vi "Lab Panel V5.0.vi"() -> ()   [LabVIEW 2013] (continued)
                        n564 = TDMS Open(6:FALSE, 10:T18."create or replace" ("operation (0:open)"), 11:w898) -> (0:w897:errorcluster, 3:→"TDMS LAB02-1":refnum<k34>)  [unwired: 4 in]
                      }
                      frame #2 {
                        n565 = local read "SET LAB02-1"() -> (w908:T5)
                        n566 = local read "TDMS LAB02-1"() -> (w919:refnum<k34>)
                        n567 = Build Array("Testers Name", "Description", "Set Test Cycles", "T-Rise minutes", "T-Rise Deg C") -> (w909:string[])
                        n568 = Unbundle(w908) -> ("NAME"=w907:string, "DESCRIPTION"=w906:string, "CYCLES"=w905:dbl, "T-RISE mins"=w904:dbl, "T-RISE deg C"=w903:dbl)
                        n569 = Number To Decimal String(number=w905) -> (decimal integer string=w918:string)  [unwired: 1 in]
                        n570 = Number To Decimal String(number=w904) -> (decimal integer string=w917:string)  [unwired: 1 in]
                        n571 = Number To Decimal String(number=w903) -> (decimal integer string=w916:string)  [unwired: 1 in]
                        n572 = Build Array(w907, w906, w918, w917, w916) -> (w915:string[])
                        n573 = TDMS Set Properties(5:w915, 7:w909, 11:w919) -> ()  [unwired: 3 in, 4 out]
                      }
                      frame #3 {
                        n574 = local read "DISP LAB02-1"() -> (w924:T4)
                        n575 = Concatenate Strings("LAB02-1  ", w923) -> (w925:string)
                        n576 = Two Button Dialog(message=w925, 1:w921, 2:w922) -> (T button?=w927:bool)
                        n577 = case shown="True" w927 {
                          tunnel: w924 -> [w934 w935]
                          tunnel: [w934 w935] -> w931
                          tunnel: [w933 w936] -> w930
                          tunnel: [w932 w936] -> w929
                          frame False {
                            n578 = Unbundle(w934) -> ("CYCLE"=w933:dbl, "MINS"=w932:dbl)  [unwired: 1 out]
                          }
                          frame True {
                            w936 = 0.0
                          }
                        }
                        n579 = Bundle(cluster=w931, "CYCLE"=w930, "MINS"=w929, "STATUS"="RUN") -> (w920:T4)
                        n580 = local write "DISP LAB02-1"(w920) -> ()
                      }
                      frame #4 {
                        n581 = local read "SIG LAB02-1"() -> (w939:T2)
                        n582 = local read "TEMP START LAB02-1"() -> (w941:cluster{"TL":dbl, "TN":dbl})
                        n583 = Unbundle(w939) -> ("Tmp Live"=w938:dbl, "Tmp Neut"=w937:dbl)  [unwired: 3 out]
                        n584 = Bundle(cluster=w941, "TL"=w938, "TN"=w937) -> (w940:cluster{"TL":dbl, "TN":dbl})
                        n585 = local write "TEMP START LAB02-1"(w940) -> ()
                      }
                    }
                  }
                }
              }
              event "RUN LAB02-2": Value Change {
                n586 = event-data() -> ("NewVal"=w945:bool)  [unwired: 1 in, 5 out]
                n587 = local write "run lab02-2"(w945) -> ()
                n588 = case shown="True" w945 {
                  tunnel: w951 -> [_ w987]
                  tunnel: w950 -> [_ w986]
                  tunnel: w948 -> [w953 w985]
                  tunnel: w949 -> [_ w984]
                  tunnel: w947 -> [_ w983]
                  tunnel: [w952 w982] -> w946
                  tunnel: w944 -> [_ w981]
                  tunnel: w943 -> [_ w980]
                  tunnel: w942 -> [_ w979]
                  frame False {
                    # "stop test"
                    n589 = stacked-sequence {
                      tunnel: w953 -> [w962 _]
                      tunnel: [w954 _] -> w952
                      frame #0 {
                        n590 = local read "DISP LAB02-2"() -> (w961:T4)
                        n591 = Unbundle(w961) -> ("CYCLE"=w959:dbl, "MINS"=w960:dbl)  [unwired: 1 out]
                        n592 = case shown="\"CYCLE TEST\"" w962 {
                          tunnel: w960 -> [_ _ w969]
                          tunnel: w959 -> [w967 w968 _]
                          tunnel: [w967 w968 w969] -> w958
                          frame "CHART TEST", Default {
                          }
                          frame "CYCLE TEST" {
                          }
                          frame "T-RISE TEST" {
                          }
                        }
                        n593 = local read "TDMS LAB02-2"() -> (w966:refnum<k34>)
                        n594 = Build Array("STOPPED") -> (w963:string[])
                        n595 = Build Array(w958) -> (w957:dbl[])
                        n596 = TDMS Write(0:w966, 5:"TEST RESULT", 7:w963, 9:w957) -> (4:w955:refnum<k34>, 15:w956:errorcluster)  [unwired: 2 in, 2 out]
                        n597 = TDMS Close(8:w956, 11:w955) -> (0:w954:errorcluster)  [unwired: 1 out]
                      }
                      frame #1 {
                        n598 = local read "DISP LAB02-2"() -> (w973:T4)
                        n599 = stacked-sequence {
                          tunnel: "LAB02-2" -> [w975 w977]
                          frame #0 {
                            n600 = call "sub vi - defrag tdms v1.vi"("panel id"=w975) -> ("error out"=w974:errorcluster)  [unwired: 10 in]
                            n601 = local write "data file error"(w974) -> ()
                          }
                          frame #1 {
                            n602 = call "Save data file to network drive v2.vi"("panel id"=w977) -> ("network file save error"=w976:errorcluster)  [unwired: 9 in, 1 out]
                            n603 = local write "RESULT LAB02-2"(FALSE) -> ()
                            n604 = local write "data file error"(w976) -> ()
                          }
                        }
                        n605 = Bundle(cluster=w973, "STATUS"="STOP") -> (w971:T4)  [unwired: 2 in]
                        n606 = local write "DISP LAB02-2"(w971) -> ()
                      }
                    }
                  }
                  frame True {
                    # "start new test and create test file"
                    n607 = stacked-sequence {
                      seq-local: [w988 _ _ _ _] -> [_ w1012 _ _ _]
                      tunnel: w987 -> [w993 _ _ _ _]
                      tunnel: w986 -> [w990 _ _ _ _]
                      tunnel: w985 -> [w1003 _ _ _ _]
                      tunnel: w984 -> [w996 _ _ _ _]
                      tunnel: w983 -> [w991 _ _ _ _]
                      tunnel: [_ w1007 _ _ _] -> w982
                      tunnel: w981 -> [_ _ _ w1033 _]
                      tunnel: w980 -> [_ _ _ w1032 _]
                      tunnel: w979 -> [_ _ _ w1031 _]
                      frame #0 {
                        w989 = "\\"
                        n608 = local read "SET LAB02-2"() -> (w998:T5)
                        n609 = case shown="\"CYCLE TEST\"" w1003 {
                          tunnel: ["L02-2-CHART TEST-" "L02-2-CYCLE TEST-" "L02-2-T-RISE TEST-"] -> w999
                          frame "CHART TEST", Default {
                          }
                          frame "CYCLE TEST" {
                          }
                          frame "T-RISE TEST" {
                          }
                        }
                        n610 = Unbundle(w998) -> ("DESCRIPTION"=w997:string)  [unwired: 4 out]
                        n611 = Concatenate Strings(w993, "\\", w991, w989, w990, w989) -> (w1000:string)
                        n612 = String To Path(string=w1000) -> (path=w1002:path)
                        n613 = Concatenate Strings(w1000, w999, w997, "-", w996, ".tdms") -> (w988:string)
                        n614 = Create Folder(path (use dialog)=w1002) -> (error out=w1001:errorcluster)  [unwired: 2 in, 2 out]
                        n615 = global write "Global 1.vi" "LAB02-2 FILE"(w988) -> ()
                        n616 = call <vilib>:"Clear Errors.vi"("error in (no error)"=w1001) -> ()  [unwired: 6 in, 1 out]
                      }
                      frame #1 {
                        (unwired) FALSE
                        n617 = String To Path(string=w1012) -> (path=w1008:path)
                        n618 = TDMS Open(6:FALSE, 10:T18."create or replace" ("operation (0:open)"), 11:w1008) -> (0:w1007:errorcluster, 3:→"TDMS LAB02-2":refnum<k34>)  [unwired: 4 in]
                      }
                      frame #2 {
                        n619 = local read "SET LAB02-2"() -> (w1018:T5)
                        n620 = local read "TDMS LAB02-2"() -> (w1029:refnum<k34>)
                        n621 = Build Array("Testers Name", "Description", "Set Test Cycles", "T-Rise minutes", "T-Rise Deg C") -> (w1019:string[])
                        n622 = Unbundle(w1018) -> ("NAME"=w1017:string, "DESCRIPTION"=w1016:string, "CYCLES"=w1015:dbl, "T-RISE mins"=w1014:dbl, "T-RISE deg C"=w1013:dbl)
                        n623 = Number To Decimal String(number=w1015) -> (decimal integer string=w1028:string)  [unwired: 1 in]
                        n624 = Number To Decimal String(number=w1014) -> (decimal integer string=w1027:string)  [unwired: 1 in]
                        n625 = Number To Decimal String(number=w1013) -> (decimal integer string=w1026:string)  [unwired: 1 in]
                        n626 = Build Array(w1017, w1016, w1028, w1027, w1026) -> (w1025:string[])
                        n627 = TDMS Set Properties(5:w1025, 7:w1019, 11:w1029) -> ()  [unwired: 3 in, 4 out]
                      }
                      frame #3 {
                        n628 = local read "DISP LAB02-2"() -> (w1034:T4)
                        n629 = Concatenate Strings("LAB02-2  ", w1033) -> (w1035:string)
                        n630 = Two Button Dialog(message=w1035, 1:w1031, 2:w1032) -> (T button?=w1037:bool)
                        n631 = case shown="True" w1037 {
                          tunnel: w1034 -> [w1044 w1045]
                          tunnel: [w1044 w1045] -> w1041
                          tunnel: [w1043 w1046] -> w1040
                          tunnel: [w1042 w1046] -> w1039
                          frame False {
                            n632 = Unbundle(w1044) -> ("CYCLE"=w1043:dbl, "MINS"=w1042:dbl)  [unwired: 1 out]
                          }
                          frame True {
                            w1046 = 0.0
                          }
                        }
                        n633 = Bundle(cluster=w1041, "CYCLE"=w1040, "MINS"=w1039, "STATUS"="RUN") -> (w1030:T4)
                        n634 = local write "DISP LAB02-2"(w1030) -> ()
                      }
                      frame #4 {
                        n635 = local read "SIG LAB02-2"() -> (w1049:T2)
                        n636 = local read "TEMP START LAB02-2"() -> (w1051:cluster{"TL":dbl, "TN":dbl})
                        n637 = Unbundle(w1049) -> ("Tmp Live"=w1048:dbl, "Tmp Neut"=w1047:dbl)  [unwired: 3 out]
                        n638 = Bundle(cluster=w1051, "TL"=w1048, "TN"=w1047) -> (w1050:cluster{"TL":dbl, "TN":dbl})
                        n639 = local write "TEMP START LAB02-2"(w1050) -> ()
                      }
                    }
                  }
                }
              }
              event "RUN LAB03-1": Value Change {
                n640 = event-data() -> ("NewVal"=w1055:bool)  [unwired: 1 in, 5 out]
                n641 = local write "run lab03-1"(w1055) -> ()
                n642 = case shown="True" w1055 {
                  tunnel: w1061 -> [_ w1097]
                  tunnel: w1060 -> [_ w1096]
                  tunnel: w1058 -> [w1063 w1095]
                  tunnel: w1059 -> [_ w1094]
                  tunnel: w1057 -> [_ w1093]
                  tunnel: [w1062 w1092] -> w1056
                  tunnel: w1054 -> [_ w1091]
                  tunnel: w1053 -> [_ w1090]
                  tunnel: w1052 -> [_ w1089]
                  frame False {
                    # "stop test"
                    n643 = stacked-sequence {
                      tunnel: w1063 -> [w1072 _]
                      tunnel: [w1064 _] -> w1062
                      frame #0 {
                        n644 = local read "DISP LAB03-1"() -> (w1071:T4)
                        n645 = Unbundle(w1071) -> ("CYCLE"=w1069:dbl, "MINS"=w1070:dbl)  [unwired: 1 out]
                        n646 = case shown="\"CYCLE TEST\"" w1072 {
                          tunnel: w1070 -> [_ _ w1079]
                          tunnel: w1069 -> [w1077 w1078 _]
                          tunnel: [w1077 w1078 w1079] -> w1068
                          frame "CHART TEST", Default {
                          }
                          frame "CYCLE TEST" {
                          }
                          frame "T-RISE TEST" {
                          }
                        }
                        n647 = local read "TDMS LAB03-1"() -> (w1076:refnum<k34>)
                        n648 = Build Array("STOPPED") -> (w1073:string[])
                        n649 = Build Array(w1068) -> (w1067:dbl[])
                        n650 = TDMS Write(0:w1076, 5:"TEST RESULT", 7:w1073, 9:w1067) -> (4:w1065:refnum<k34>, 15:w1066:errorcluster)  [unwired: 2 in, 2 out]
                        n651 = TDMS Close(8:w1066, 11:w1065) -> (0:w1064:errorcluster)  [unwired: 1 out]
                      }
                      frame #1 {
                        n652 = local read "DISP LAB03-1"() -> (w1083:T4)
                        n653 = stacked-sequence {
                          tunnel: "LAB03-1" -> [w1085 w1087]
                          frame #0 {
                            n654 = call "sub vi - defrag tdms v1.vi"("panel id"=w1085) -> ("error out"=w1084:errorcluster)  [unwired: 10 in]
                            n655 = local write "data file error"(w1084) -> ()
                          }
                          frame #1 {
                            n656 = call "Save data file to network drive v2.vi"("panel id"=w1087) -> ("network file save error"=w1086:errorcluster)  [unwired: 9 in, 1 out]
                            n657 = local write "RESULT LAB03-1"(FALSE) -> ()
                            n658 = local write "data file error"(w1086) -> ()
                          }
                        }
                        n659 = Bundle(cluster=w1083, "STATUS"="STOP") -> (w1081:T4)  [unwired: 2 in]
                        n660 = local write "DISP LAB03-1"(w1081) -> ()
                      }
                    }
                  }
                  frame True {
                    # "start new test and create test file"
                    n661 = stacked-sequence {
                      seq-local: [w1098 _ _ _ _] -> [_ w1122 _ _ _]
                      tunnel: w1097 -> [w1103 _ _ _ _]
                      tunnel: w1096 -> [w1100 _ _ _ _]
                      tunnel: w1095 -> [w1113 _ _ _ _]
                      tunnel: w1094 -> [w1106 _ _ _ _]
                      tunnel: w1093 -> [w1101 _ _ _ _]
                      tunnel: [_ w1117 _ _ _] -> w1092
                      tunnel: w1091 -> [_ _ _ w1142 _]
                      tunnel: w1090 -> [_ _ _ w1141 _]
                      tunnel: w1089 -> [_ _ _ w1140 _]
                      frame #0 {
                        w1099 = "\\"
                        n662 = local read "SET LAB03-1"() -> (w1108:T5)
                        n663 = case shown="\"T-RISE TEST\"" w1113 {
                          tunnel: ["L03-1-CHART TEST-" "L03-1-CYCLE TEST-" "L03-1-T-RISE TEST-"] -> w1109
                          frame "CHART TEST", Default {
                          }
                          frame "CYCLE TEST" {
                          }
                          frame "T-RISE TEST" {
                          }
                        }
                        n664 = Unbundle(w1108) -> ("DESCRIPTION"=w1107:string)  [unwired: 4 out]
                        n665 = Concatenate Strings(w1103, "\\", w1101, w1099, w1100, w1099) -> (w1110:string)
                        n666 = String To Path(string=w1110) -> (path=w1112:path)
                        n667 = Concatenate Strings(w1110, w1109, w1107, "-", w1106, ".tdms") -> (w1098:string)
                        n668 = Create Folder(path (use dialog)=w1112) -> (error out=w1111:errorcluster)  [unwired: 2 in, 2 out]
                        n669 = global write "Global 1.vi" "LAB03-1 FILE"(w1098) -> ()
                        n670 = call <vilib>:"Clear Errors.vi"("error in (no error)"=w1111) -> ()  [unwired: 6 in, 1 out]
                      }
                      frame #1 {
                        (unwired) FALSE
                        n671 = String To Path(string=w1122) -> (path=w1118:path)
                        n672 = TDMS Open(6:FALSE, 10:T18."create or replace" ("operation (0:open)"), 11:w1118) -> (0:w1117:errorcluster, 3:→"TDMS LAB03-1":refnum<k34>)  [unwired: 4 in]
                      }
                      frame #2 {
                        n673 = local read "SET LAB03-1"() -> (w1128:T5)
                        n674 = local read "TDMS LAB03-1"() -> (w1139:refnum<k34>)
                        n675 = Build Array("Testers Name", "Description", "Set Test Cycles", "T-Rise minutes", "T-Rise Deg C") -> (w1129:string[])
                        n676 = Unbundle(w1128) -> ("NAME"=w1127:string, "DESCRIPTION"=w1126:string, "CYCLES"=w1125:dbl, "T-RISE mins"=w1124:dbl, "T-RISE deg C"=w1123:dbl)
                        n677 = Number To Decimal String(number=w1125) -> (decimal integer string=w1138:string)  [unwired: 1 in]
                        n678 = Number To Decimal String(number=w1124) -> (decimal integer string=w1137:string)  [unwired: 1 in]
                        n679 = Number To Decimal String(number=w1123) -> (decimal integer string=w1136:string)  [unwired: 1 in]
                        n680 = Build Array(w1127, w1126, w1138, w1137, w1136) -> (w1135:string[])
                        n681 = TDMS Set Properties(5:w1135, 7:w1129, 11:w1139) -> ()  [unwired: 3 in, 4 out]
                      }
                      frame #3 {
                        n682 = local read "DISP LAB03-1"() -> (w1144:T4)
                        n683 = Concatenate Strings("LAB03-1  ", w1142) -> (w1145:string)
                        n684 = Two Button Dialog(message=w1145, 1:w1140, 2:w1141) -> (T button?=w1147:bool)
                        n685 = case shown="True" w1147 {
                          tunnel: w1144 -> [w1154 w1155]
                          tunnel: [w1154 w1155] -> w1151
                          tunnel: [w1153 w1156] -> w1150
                          tunnel: [w1152 w1156] -> w1149
                          frame False {
                            n686 = Unbundle(w1154) -> ("CYCLE"=w1153:dbl, "MINS"=w1152:dbl)  [unwired: 1 out]
                          }
                          frame True {
                            w1156 = 0.0
                          }
                        }
                        n687 = Bundle(cluster=w1151, "CYCLE"=w1150, "MINS"=w1149, "STATUS"="RUN") -> (w1143:T4)
                        n688 = local write "DISP LAB03-1"(w1143) -> ()
                      }
                      frame #4 {
                        n689 = local read "SIG LAB03-1"() -> (w1159:T2)
                        n690 = local read "TEMP START LAB03-1"() -> (w1161:cluster{"TL":dbl, "TN":dbl})
                        n691 = Unbundle(w1159) -> ("Tmp Live"=w1158:dbl, "Tmp Neut"=w1157:dbl)  [unwired: 3 out]
                        n692 = Bundle(cluster=w1161, "TL"=w1158, "TN"=w1157) -> (w1160:cluster{"TL":dbl, "TN":dbl})
                        n693 = local write "TEMP START LAB03-1"(w1160) -> ()
                      }
                    }
                  }
                }
              }
              event "RUN LAB03-2": Value Change {
                n694 = event-data() -> ("NewVal"=w1165:bool)  [unwired: 1 in, 5 out]
                n695 = local write "run lab03-2"(w1165) -> ()
                n696 = case shown="True" w1165 {
                  tunnel: w1171 -> [_ w1207]
                  tunnel: w1170 -> [_ w1206]
                  tunnel: w1168 -> [w1173 w1205]
                  tunnel: w1169 -> [_ w1204]
                  tunnel: w1167 -> [_ w1203]
                  tunnel: [w1172 w1202] -> w1166
                  tunnel: w1164 -> [_ w1201]
                  tunnel: w1163 -> [_ w1200]
                  tunnel: w1162 -> [_ w1199]
                  frame False {
                    # "stop test"
                    n697 = stacked-sequence {
                      tunnel: w1173 -> [w1182 _]
                      tunnel: [w1174 _] -> w1172
                      frame #0 {
                        n698 = local read "DISP LAB03-2"() -> (w1181:T4)
                        n699 = Unbundle(w1181) -> ("CYCLE"=w1179:dbl, "MINS"=w1180:dbl)  [unwired: 1 out]
                        n700 = case shown="\"CYCLE TEST\"" w1182 {
                          tunnel: w1180 -> [_ _ w1189]
                          tunnel: w1179 -> [w1187 w1188 _]
                          tunnel: [w1187 w1188 w1189] -> w1178
                          frame "CHART TEST", Default {
                          }
                          frame "CYCLE TEST" {
                          }
                          frame "T-RISE TEST" {
                          }
                        }
                        n701 = local read "TDMS LAB03-2"() -> (w1186:refnum<k34>)
                        n702 = Build Array("STOPPED") -> (w1183:string[])
                        n703 = Build Array(w1178) -> (w1177:dbl[])
                        n704 = TDMS Write(0:w1186, 5:"TEST RESULT", 7:w1183, 9:w1177) -> (4:w1175:refnum<k34>, 15:w1176:errorcluster)  [unwired: 2 in, 2 out]
                        n705 = TDMS Close(8:w1176, 11:w1175) -> (0:w1174:errorcluster)  [unwired: 1 out]
                      }
                      frame #1 {
                        n706 = local read "DISP LAB03-2"() -> (w1193:T4)
                        n707 = stacked-sequence {
                          tunnel: "LAB03-2" -> [w1195 w1197]
                          frame #0 {
                            n708 = call "sub vi - defrag tdms v1.vi"("panel id"=w1195) -> ("error out"=w1194:errorcluster)  [unwired: 10 in]
                            n709 = local write "data file error"(w1194) -> ()
                          }
                          frame #1 {
                            n710 = call "Save data file to network drive v2.vi"("panel id"=w1197) -> ("network file save error"=w1196:errorcluster)  [unwired: 9 in, 1 out]
                            n711 = local write "RESULT LAB03-2"(FALSE) -> ()
                            n712 = local write "data file error"(w1196) -> ()
                          }
                        }
                        n713 = Bundle(cluster=w1193, "STATUS"="STOP") -> (w1191:T4)  [unwired: 2 in]
                        n714 = local write "DISP LAB03-2"(w1191) -> ()
                      }
                    }
                  }
                  frame True {
                    # "start new test and create test file"
                    n715 = stacked-sequence {
                      seq-local: [w1208 _ _ _ _] -> [_ w1232 _ _ _]
                      tunnel: w1207 -> [w1213 _ _ _ _]
                      tunnel: w1206 -> [w1210 _ _ _ _]
                      tunnel: w1205 -> [w1223 _ _ _ _]
                      tunnel: w1204 -> [w1216 _ _ _ _]
                      tunnel: w1203 -> [w1211 _ _ _ _]
                      tunnel: [_ w1227 _ _ _] -> w1202
                      tunnel: w1201 -> [_ _ _ w1253 _]
                      tunnel: w1200 -> [_ _ _ w1252 _]
                      tunnel: w1199 -> [_ _ _ w1251 _]
                      frame #0 {
                        w1209 = "\\"
                        n716 = local read "SET LAB03-2"() -> (w1218:T5)
                        n717 = case shown="\"T-RISE TEST\"" w1223 {
                          tunnel: ["L03-2-CHART TEST-" "L03-2-CYCLE TEST-" "L03-2-T-RISE TEST-"] -> w1219
                          frame "CHART TEST", Default {
                          }
                          frame "CYCLE TEST" {
                          }
                          frame "T-RISE TEST" {
                          }
                        }
                        n718 = Unbundle(w1218) -> ("DESCRIPTION"=w1217:string)  [unwired: 4 out]
                        n719 = Concatenate Strings(w1213, "\\", w1211, w1209, w1210, w1209) -> (w1220:string)
                        n720 = String To Path(string=w1220) -> (path=w1222:path)
                        n721 = Concatenate Strings(w1220, w1219, w1217, "-", w1216, ".tdms") -> (w1208:string)
                        n722 = Create Folder(path (use dialog)=w1222) -> (error out=w1221:errorcluster)  [unwired: 2 in, 2 out]
                        n723 = global write "Global 1.vi" "LAB03-2 FILE"(w1208) -> ()
                        n724 = call <vilib>:"Clear Errors.vi"("error in (no error)"=w1221) -> ()  [unwired: 6 in, 1 out]
                      }
                      frame #1 {
                        (unwired) FALSE
                        n725 = String To Path(string=w1232) -> (path=w1228:path)
                        n726 = TDMS Open(6:FALSE, 10:T18."create or replace" ("operation (0:open)"), 11:w1228) -> (0:w1227:errorcluster, 3:→"TDMS LAB03-2":refnum<k34>)  [unwired: 4 in]
                      }
                      frame #2 {
                        n727 = local read "SET LAB03-2"() -> (w1238:T5)
                        n728 = local read "TDMS LAB03-2"() -> (w1249:refnum<k34>)
                        n729 = Build Array("Testers Name", "Description", "Set Test Cycles", "T-Rise minutes", "T-Rise Deg C") -> (w1239:string[])
                        n730 = Unbundle(w1238) -> ("NAME"=w1237:string, "DESCRIPTION"=w1236:string, "CYCLES"=w1235:dbl, "T-RISE mins"=w1234:dbl, "T-RISE deg C"=w1233:dbl)
                        n731 = Number To Decimal String(number=w1235) -> (decimal integer string=w1248:string)  [unwired: 1 in]
                        n732 = Number To Decimal String(number=w1234) -> (decimal integer string=w1247:string)  [unwired: 1 in]
                        n733 = Number To Decimal String(number=w1233) -> (decimal integer string=w1246:string)  [unwired: 1 in]
                        n734 = Build Array(w1237, w1236, w1248, w1247, w1246) -> (w1245:string[])
                        n735 = TDMS Set Properties(5:w1245, 7:w1239, 11:w1249) -> ()  [unwired: 3 in, 4 out]
                      }
                      frame #3 {
                        n736 = local read "DISP LAB03-2"() -> (w1254:T4)
                        n737 = Concatenate Strings("LAB03-2  ", w1253) -> (w1255:string)
                        n738 = Two Button Dialog(message=w1255, 1:w1251, 2:w1252) -> (T button?=w1257:bool)
                        n739 = case shown="True" w1257 {
                          tunnel: w1254 -> [w1264 w1265]
                          tunnel: [w1264 w1265] -> w1261
                          tunnel: [w1263 w1266] -> w1260
                          tunnel: [w1262 w1266] -> w1259
                          frame False {
                            n740 = Unbundle(w1264) -> ("CYCLE"=w1263:dbl, "MINS"=w1262:dbl)  [unwired: 1 out]
                          }
                          frame True {
                            w1266 = 0.0
                          }
                        }
                        n741 = Bundle(cluster=w1261, "CYCLE"=w1260, "MINS"=w1259, "STATUS"="RUN") -> (w1250:T4)
                        n742 = local write "DISP LAB03-2"(w1250) -> ()
                      }
                      frame #4 {
                        n743 = local read "SIG LAB03-2"() -> (w1269:T2)
                        n744 = local read "TEMP START LAB03-2"() -> (w1271:cluster{"TL":dbl, "TN":dbl})
                        n745 = Unbundle(w1269) -> ("Tmp Live"=w1268:dbl, "Tmp Neut"=w1267:dbl)  [unwired: 3 out]
                        n746 = Bundle(cluster=w1271, "TL"=w1268, "TN"=w1267) -> (w1270:cluster{"TL":dbl, "TN":dbl})
                        n747 = local write "TEMP START LAB03-2"(w1270) -> ()
                      }
                    }
                  }
                }
              }
              event "RUN LAB04-1": Value Change {
                n748 = event-data() -> ("NewVal"=w1275:bool)  [unwired: 1 in, 5 out]
                n749 = local write "run lab04-1"(w1275) -> ()
                n750 = case shown="True" w1275 {
                  tunnel: w1281 -> [_ w1317]
                  tunnel: w1280 -> [_ w1316]
                  tunnel: w1278 -> [w1283 w1315]
                  tunnel: w1279 -> [_ w1314]
                  tunnel: w1277 -> [_ w1313]
                  tunnel: [w1282 w1312] -> w1276
                  tunnel: w1274 -> [_ w1311]
                  tunnel: w1273 -> [_ w1310]
                  tunnel: w1272 -> [_ w1309]
                  frame False {
                    # "stop test"
                    n751 = stacked-sequence {
                      tunnel: w1283 -> [w1292 _]
                      tunnel: [w1284 _] -> w1282
                      frame #0 {
                        n752 = local read "DISP LAB04-1"() -> (w1291:T4)
                        n753 = Unbundle(w1291) -> ("CYCLE"=w1289:dbl, "MINS"=w1290:dbl)  [unwired: 1 out]
                        n754 = case shown="\"CYCLE TEST\"" w1292 {
                          tunnel: w1290 -> [_ _ w1299]
                          tunnel: w1289 -> [w1297 w1298 _]
                          tunnel: [w1297 w1298 w1299] -> w1288
                          frame "CHART TEST", Default {
                          }
                          frame "CYCLE TEST" {
                          }
                          frame "T-RISE TEST" {
                          }
                        }
                        n755 = local read "TDMS LAB04-1"() -> (w1296:refnum<k34>)
                        n756 = Build Array("STOPPED") -> (w1293:string[])
                        n757 = Build Array(w1288) -> (w1287:dbl[])
                        n758 = TDMS Write(0:w1296, 5:"TEST RESULT", 7:w1293, 9:w1287) -> (4:w1285:refnum<k34>, 15:w1286:errorcluster)  [unwired: 2 in, 2 out]
                        n759 = TDMS Close(8:w1286, 11:w1285) -> (0:w1284:errorcluster)  [unwired: 1 out]
                      }
                      frame #1 {
                        n760 = local read "DISP LAB04-1"() -> (w1303:T4)
                        n761 = stacked-sequence {
                          tunnel: "LAB04-1" -> [w1305 w1307]
                          frame #0 {
                            n762 = call "sub vi - defrag tdms v1.vi"("panel id"=w1305) -> ("error out"=w1304:errorcluster)  [unwired: 10 in]
                            n763 = local write "data file error"(w1304) -> ()
                          }
                          frame #1 {
                            n764 = call "Save data file to network drive v2.vi"("panel id"=w1307) -> ("network file save error"=w1306:errorcluster)  [unwired: 9 in, 1 out]
                            n765 = local write "RESULT LAB04-1"(FALSE) -> ()
                            n766 = local write "data file error"(w1306) -> ()
                          }
                        }
                        n767 = Bundle(cluster=w1303, "STATUS"="STOP") -> (w1301:T4)  [unwired: 2 in]
                        n768 = local write "DISP LAB04-1"(w1301) -> ()
                      }
                    }
                  }
                  frame True {
                    # "start new test and create test file"
                    n769 = stacked-sequence {
                      seq-local: [w1318 _ _ _ _] -> [_ w1342 _ _ _]
                      tunnel: w1317 -> [w1323 _ _ _ _]
                      tunnel: w1316 -> [w1319 _ _ _ _]
                      tunnel: w1315 -> [w1333 _ _ _ _]
                      tunnel: w1314 -> [w1326 _ _ _ _]
                      tunnel: w1313 -> [w1321 _ _ _ _]
                      tunnel: [_ w1337 _ _ _] -> w1312
                      tunnel: w1311 -> [_ _ _ w1363 _]
                      tunnel: w1310 -> [_ _ _ w1362 _]
                      tunnel: w1309 -> [_ _ _ w1361 _]
                      frame #0 {
                        w1320 = "\\"
                        n770 = local read "SET LAB04-1"() -> (w1328:T5)
                        n771 = case shown="\"CYCLE TEST\"" w1333 {
                          tunnel: ["L04-1-CHART TEST-" "L04-1-CYCLE TEST-" "L04-1-T-RISE TEST-"] -> w1329
                          frame "CHART TEST", Default {
                          }
                          frame "CYCLE TEST" {
                          }
                          frame "T-RISE TEST" {
                          }
                        }
                        n772 = Unbundle(w1328) -> ("DESCRIPTION"=w1327:string)  [unwired: 4 out]
                        n773 = Concatenate Strings(w1323, "\\", w1321, w1320, w1319, w1320) -> (w1330:string)
                        n774 = String To Path(string=w1330) -> (path=w1332:path)
                        n775 = Concatenate Strings(w1330, w1329, w1327, "-", w1326, ".tdms") -> (w1318:string)
                        n776 = Create Folder(path (use dialog)=w1332) -> (error out=w1331:errorcluster)  [unwired: 2 in, 2 out]
                        n777 = global write "Global 1.vi" "LAB04-1 FILE"(w1318) -> ()
                        n778 = call <vilib>:"Clear Errors.vi"("error in (no error)"=w1331) -> ()  [unwired: 6 in, 1 out]
                      }
                      frame #1 {
                        (unwired) FALSE
                        n779 = String To Path(string=w1342) -> (path=w1338:path)
                        n780 = TDMS Open(6:FALSE, 10:T18."create or replace" ("operation (0:open)"), 11:w1338) -> (0:w1337:errorcluster, 3:→"TDMS LAB04-1":refnum<k34>)  [unwired: 4 in]
                      }
                      frame #2 {
                        n781 = local read "SET LAB04-1"() -> (w1348:T5)
                        n782 = local read "TDMS LAB04-1"() -> (w1359:refnum<k34>)
                        n783 = Build Array("Testers Name", "Description", "Set Test Cycles", "T-Rise minutes", "T-Rise Deg C") -> (w1349:string[])
                        n784 = Unbundle(w1348) -> ("NAME"=w1347:string, "DESCRIPTION"=w1346:string, "CYCLES"=w1345:dbl, "T-RISE mins"=w1344:dbl, "T-RISE deg C"=w1343:dbl)
                        n785 = Number To Decimal String(number=w1345) -> (decimal integer string=w1358:string)  [unwired: 1 in]
                        n786 = Number To Decimal String(number=w1344) -> (decimal integer string=w1357:string)  [unwired: 1 in]
                        n787 = Number To Decimal String(number=w1343) -> (decimal integer string=w1356:string)  [unwired: 1 in]
                        n788 = Build Array(w1347, w1346, w1358, w1357, w1356) -> (w1355:string[])
                        n789 = TDMS Set Properties(5:w1355, 7:w1349, 11:w1359) -> ()  [unwired: 3 in, 4 out]
                      }
                      frame #3 {
                        n790 = local read "DISP LAB04-1"() -> (w1364:T4)
                        n791 = Concatenate Strings("LAB04-1  ", w1363) -> (w1365:string)
                        n792 = Two Button Dialog(message=w1365, 1:w1361, 2:w1362) -> (T button?=w1367:bool)
                        n793 = case shown="True" w1367 {
                          tunnel: w1364 -> [w1374 w1375]
                          tunnel: [w1374 w1375] -> w1371
                          tunnel: [w1373 w1376] -> w1370
                          tunnel: [w1372 w1376] -> w1369
                          frame False {
                            n794 = Unbundle(w1374) -> ("CYCLE"=w1373:dbl, "MINS"=w1372:dbl)  [unwired: 1 out]
                          }
                          frame True {
                            w1376 = 0.0
                          }
                        }
                        n795 = Bundle(cluster=w1371, "CYCLE"=w1370, "MINS"=w1369, "STATUS"="RUN") -> (w1360:T4)
                        n796 = local write "DISP LAB04-1"(w1360) -> ()
                      }
                      frame #4 {
                        n797 = local read "SIG LAB04-1"() -> (w1379:T2)
                        n798 = local read "TEMP START LAB04-1"() -> (w1381:cluster{"TL":dbl, "TN":dbl})
                        n799 = Unbundle(w1379) -> ("Tmp Live"=w1378:dbl, "Tmp Neut"=w1377:dbl)  [unwired: 3 out]
                        n800 = Bundle(cluster=w1381, "TL"=w1378, "TN"=w1377) -> (w1380:cluster{"TL":dbl, "TN":dbl})
                        n801 = local write "TEMP START LAB04-1"(w1380) -> ()
                      }
                    }
                  }
                }
              }
              event "RUN LAB04-2": Value Change {
                n802 = event-data() -> ("NewVal"=w1385:bool)  [unwired: 1 in, 5 out]
                n803 = local write "run lab04-2"(w1385) -> ()
                n804 = case shown="True" w1385 {
                  tunnel: w1391 -> [_ w1427]
                  tunnel: w1390 -> [_ w1426]
                  tunnel: w1388 -> [w1393 w1425]
                  tunnel: w1389 -> [_ w1424]
                  tunnel: w1387 -> [_ w1423]
                  tunnel: [w1392 w1422] -> w1386
                  tunnel: w1384 -> [_ w1421]
                  tunnel: w1383 -> [_ w1420]
                  tunnel: w1382 -> [_ w1419]
                  frame False {
                    # "stop test"
                    n805 = stacked-sequence {
                      tunnel: w1393 -> [w1402 _]
                      tunnel: [w1394 _] -> w1392
                      frame #0 {
                        n806 = local read "DISP LAB04-2"() -> (w1401:T4)
                        n807 = Unbundle(w1401) -> ("CYCLE"=w1399:dbl, "MINS"=w1400:dbl)  [unwired: 1 out]
                        n808 = case shown="\"CYCLE TEST\"" w1402 {
                          tunnel: w1400 -> [_ _ w1409]
                          tunnel: w1399 -> [w1407 w1408 _]
                          tunnel: [w1407 w1408 w1409] -> w1398
                          frame "CHART TEST", Default {
                          }
                          frame "CYCLE TEST" {
                          }
                          frame "T-RISE TEST" {
                          }
                        }
                        n809 = local read "TDMS LAB04-2"() -> (w1406:refnum<k34>)
                        n810 = Build Array("STOPPED") -> (w1403:string[])
                        n811 = Build Array(w1398) -> (w1397:dbl[])
                        n812 = TDMS Write(0:w1406, 5:"TEST RESULT", 7:w1403, 9:w1397) -> (4:w1395:refnum<k34>, 15:w1396:errorcluster)  [unwired: 2 in, 2 out]
                        n813 = TDMS Close(8:w1396, 11:w1395) -> (0:w1394:errorcluster)  [unwired: 1 out]
                      }
                      frame #1 {
                        n814 = local read "DISP LAB04-2"() -> (w1413:T4)
                        n815 = stacked-sequence {
                          tunnel: "LAB04-2" -> [w1415 w1417]
                          frame #0 {
                            n816 = call "sub vi - defrag tdms v1.vi"("panel id"=w1415) -> ("error out"=w1414:errorcluster)  [unwired: 10 in]
                            n817 = local write "data file error"(w1414) -> ()
                          }
                          frame #1 {
                            n818 = call "Save data file to network drive v2.vi"("panel id"=w1417) -> ("network file save error"=w1416:errorcluster)  [unwired: 9 in, 1 out]
                            n819 = local write "RESULT LAB04-2"(FALSE) -> ()
                            n820 = local write "data file error"(w1416) -> ()
                          }
                        }
                        n821 = Bundle(cluster=w1413, "STATUS"="STOP") -> (w1411:T4)  [unwired: 2 in]
                        n822 = local write "DISP LAB04-2"(w1411) -> ()
                      }
                    }
                  }
                  frame True {
                    # "start new test and create test file"
                    n823 = stacked-sequence {
                      seq-local: [w1428 _ _ _ _] -> [_ w1452 _ _ _]
                      tunnel: w1427 -> [w1433 _ _ _ _]
                      tunnel: w1426 -> [w1429 _ _ _ _]
                      tunnel: w1425 -> [w1443 _ _ _ _]
                      tunnel: w1424 -> [w1436 _ _ _ _]
                      tunnel: w1423 -> [w1431 _ _ _ _]
                      tunnel: [_ w1447 _ _ _] -> w1422
                      tunnel: w1421 -> [_ _ _ w1473 _]
                      tunnel: w1420 -> [_ _ _ w1472 _]
                      tunnel: w1419 -> [_ _ _ w1471 _]
                      frame #0 {
                        w1430 = "\\"
                        n824 = local read "SET LAB04-2"() -> (w1438:T5)
                        n825 = case shown="\"CHART TEST\", Default" w1443 {
                          tunnel: ["L04-2-CHART TEST-" "L04-2-CYCLE TEST-" "L04-2-T-RISE TEST-"] -> w1439
                          frame "CHART TEST", Default {
                          }
                          frame "CYCLE TEST" {
                          }
                          frame "T-RISE TEST" {
                          }
                        }
                        n826 = Unbundle(w1438) -> ("DESCRIPTION"=w1437:string)  [unwired: 4 out]
                        n827 = Concatenate Strings(w1433, "\\", w1431, w1430, w1429, w1430) -> (w1440:string)
                        n828 = String To Path(string=w1440) -> (path=w1442:path)
                        n829 = Concatenate Strings(w1440, w1439, w1437, "-", w1436, ".tdms") -> (w1428:string)
                        n830 = Create Folder(path (use dialog)=w1442) -> (error out=w1441:errorcluster)  [unwired: 2 in, 2 out]
                        n831 = global write "Global 1.vi" "LAB04-2 FILE"(w1428) -> ()
                        n832 = call <vilib>:"Clear Errors.vi"("error in (no error)"=w1441) -> ()  [unwired: 6 in, 1 out]
                      }
                      frame #1 {
                        (unwired) FALSE
                        n833 = String To Path(string=w1452) -> (path=w1448:path)
                        n834 = TDMS Open(6:FALSE, 10:T18."create or replace" ("operation (0:open)"), 11:w1448) -> (0:w1447:errorcluster, 3:→"TDMS LAB04-2":refnum<k34>)  [unwired: 4 in]
                      }
                      frame #2 {
                        n835 = local read "SET LAB04-2"() -> (w1458:T5)
                        n836 = local read "TDMS LAB04-2"() -> (w1469:refnum<k34>)
                        n837 = Build Array("Testers Name", "Description", "Set Test Cycles", "T-Rise minutes", "T-Rise Deg C") -> (w1459:string[])
                        n838 = Unbundle(w1458) -> ("NAME"=w1457:string, "DESCRIPTION"=w1456:string, "CYCLES"=w1455:dbl, "T-RISE mins"=w1454:dbl, "T-RISE deg C"=w1453:dbl)
                        n839 = Number To Decimal String(number=w1455) -> (decimal integer string=w1468:string)  [unwired: 1 in]
                        n840 = Number To Decimal String(number=w1454) -> (decimal integer string=w1467:string)  [unwired: 1 in]
                        n841 = Number To Decimal String(number=w1453) -> (decimal integer string=w1466:string)  [unwired: 1 in]
                        n842 = Build Array(w1457, w1456, w1468, w1467, w1466) -> (w1465:string[])
                        n843 = TDMS Set Properties(5:w1465, 7:w1459, 11:w1469) -> ()  [unwired: 3 in, 4 out]
                      }
                      frame #3 {
                        n844 = local read "DISP LAB04-2"() -> (w1474:T4)
                        n845 = Concatenate Strings("LAB04-2 ", w1473) -> (w1475:string)
                        n846 = Two Button Dialog(message=w1475, 1:w1471, 2:w1472) -> (T button?=w1477:bool)
                        n847 = case shown="True" w1477 {
                          tunnel: w1474 -> [w1484 w1485]
                          tunnel: [w1484 w1485] -> w1481
                          tunnel: [w1483 w1486] -> w1480
                          tunnel: [w1482 w1486] -> w1479
                          frame False {
                            n848 = Unbundle(w1484) -> ("CYCLE"=w1483:dbl, "MINS"=w1482:dbl)  [unwired: 1 out]
                          }
                          frame True {
                            w1486 = 0.0
                          }
                        }
                        n849 = Bundle(cluster=w1481, "CYCLE"=w1480, "MINS"=w1479, "STATUS"="RUN") -> (w1470:T4)
                        n850 = local write "DISP LAB04-2"(w1470) -> ()
                      }
                      frame #4 {
                        n851 = local read "SIG LAB04-2"() -> (w1489:T2)
                        n852 = local read "TEMP START LAB04-2"() -> (w1491:cluster{"TL":dbl, "TN":dbl})
                        n853 = Unbundle(w1489) -> ("Tmp Live"=w1488:dbl, "Tmp Neut"=w1487:dbl)  [unwired: 3 out]
                        n854 = Bundle(cluster=w1491, "TL"=w1488, "TN"=w1487) -> (w1490:cluster{"TL":dbl, "TN":dbl})
                        n855 = local write "TEMP START LAB04-2"(w1490) -> ()
                      }
                    }
                  }
                }
              }
              event "RUN LAB05-1": Value Change {
                n856 = event-data() -> ("NewVal"=w1495:bool)  [unwired: 1 in, 5 out]
                n857 = local write "run lab05-1"(w1495) -> ()
                n858 = case shown="True" w1495 {
                  tunnel: w1501 -> [_ w1537]
                  tunnel: w1500 -> [_ w1536]
                  tunnel: w1498 -> [w1503 w1535]
                  tunnel: w1499 -> [_ w1534]
                  tunnel: w1497 -> [_ w1533]
                  tunnel: [w1502 w1532] -> w1496
                  tunnel: w1494 -> [_ w1531]
                  tunnel: w1493 -> [_ w1530]
                  tunnel: w1492 -> [_ w1529]
                  frame False {
                    # "stop test"
                    n859 = stacked-sequence {
                      tunnel: w1503 -> [w1512 _]
                      tunnel: [w1504 _] -> w1502
                      frame #0 {
                        n860 = local read "DISP LAB05-1"() -> (w1511:T4)
                        n861 = Unbundle(w1511) -> ("CYCLE"=w1509:dbl, "MINS"=w1510:dbl)  [unwired: 1 out]
                        n862 = case shown="\"CYCLE TEST\"" w1512 {
                          tunnel: w1510 -> [_ _ w1519]
                          tunnel: w1509 -> [w1517 w1518 _]
                          tunnel: [w1517 w1518 w1519] -> w1508
                          frame "CHART TEST", Default {
                          }
                          frame "CYCLE TEST" {
                          }
                          frame "T-RISE TEST" {
                          }
                        }
                        n863 = local read "TDMS LAB05-1"() -> (w1516:refnum<k34>)
                        n864 = Build Array("STOPPED") -> (w1513:string[])
                        n865 = Build Array(w1508) -> (w1507:dbl[])
                        n866 = TDMS Write(0:w1516, 5:"TEST RESULT", 7:w1513, 9:w1507) -> (4:w1505:refnum<k34>, 15:w1506:errorcluster)  [unwired: 2 in, 2 out]
                        n867 = TDMS Close(8:w1506, 11:w1505) -> (0:w1504:errorcluster)  [unwired: 1 out]
                      }
                      frame #1 {
                        n868 = local read "DISP LAB05-1"() -> (w1523:T4)
                        n869 = stacked-sequence {
                          tunnel: "LAB05-1" -> [w1525 w1527]
                          frame #0 {
                            n870 = call "sub vi - defrag tdms v1.vi"("panel id"=w1525) -> ("error out"=w1524:errorcluster)  [unwired: 10 in]
                            n871 = local write "data file error"(w1524) -> ()
                          }
                          frame #1 {
                            n872 = call "Save data file to network drive v2.vi"("panel id"=w1527) -> ("network file save error"=w1526:errorcluster)  [unwired: 9 in, 1 out]
                            n873 = local write "RESULT LAB05-1"(FALSE) -> ()
                            n874 = local write "data file error"(w1526) -> ()
                          }
                        }
                        n875 = Bundle(cluster=w1523, "STATUS"="STOP") -> (w1521:T4)  [unwired: 2 in]
                        n876 = local write "DISP LAB05-1"(w1521) -> ()
                      }
                    }
                  }
                  frame True {
                    # "start new test and create test file"
                    n877 = stacked-sequence {
                      seq-local: [w1538 _ _ _ _] -> [_ w1562 _ _ _]
                      tunnel: w1537 -> [w1543 _ _ _ _]
                      tunnel: w1536 -> [w1539 _ _ _ _]
                      tunnel: w1535 -> [w1553 _ _ _ _]
                      tunnel: w1534 -> [w1546 _ _ _ _]
                      tunnel: w1533 -> [w1541 _ _ _ _]
                      tunnel: [_ w1557 _ _ _] -> w1532
                      tunnel: w1531 -> [_ _ _ w1582 _]
                      tunnel: w1530 -> [_ _ _ w1581 _]
                      tunnel: w1529 -> [_ _ _ w1580 _]
                      frame #0 {
